vi "RT-v.vi"() -> ()   [LabVIEW 2013]
uses:
  FreqEstimator.ctl
panel:
  out "theta":sgl(graph)
  in  "Scaling":sgl
  in  "alpha":sgl
  in  "Input":sgl
  in  "stop":bool
  in  "Frequency of Oscillation":sgl
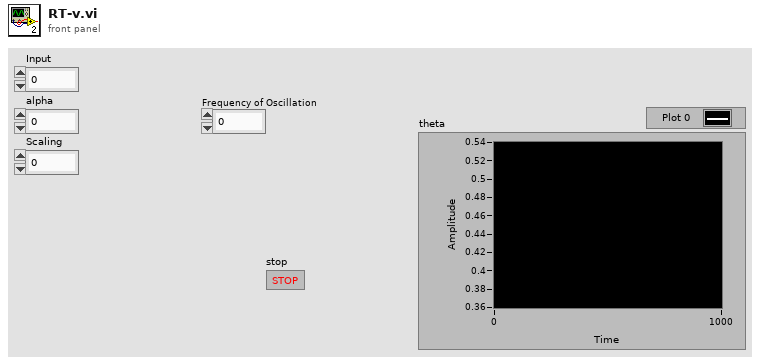
[diagram p1: front panel]
types:
  T1 = typedef "FreqEstimator.ctl" = cluster{"Parameters":cluster{"Ts":sgl, "kappaav":sgl, "kappaph":sgl, "mu":sgl}}
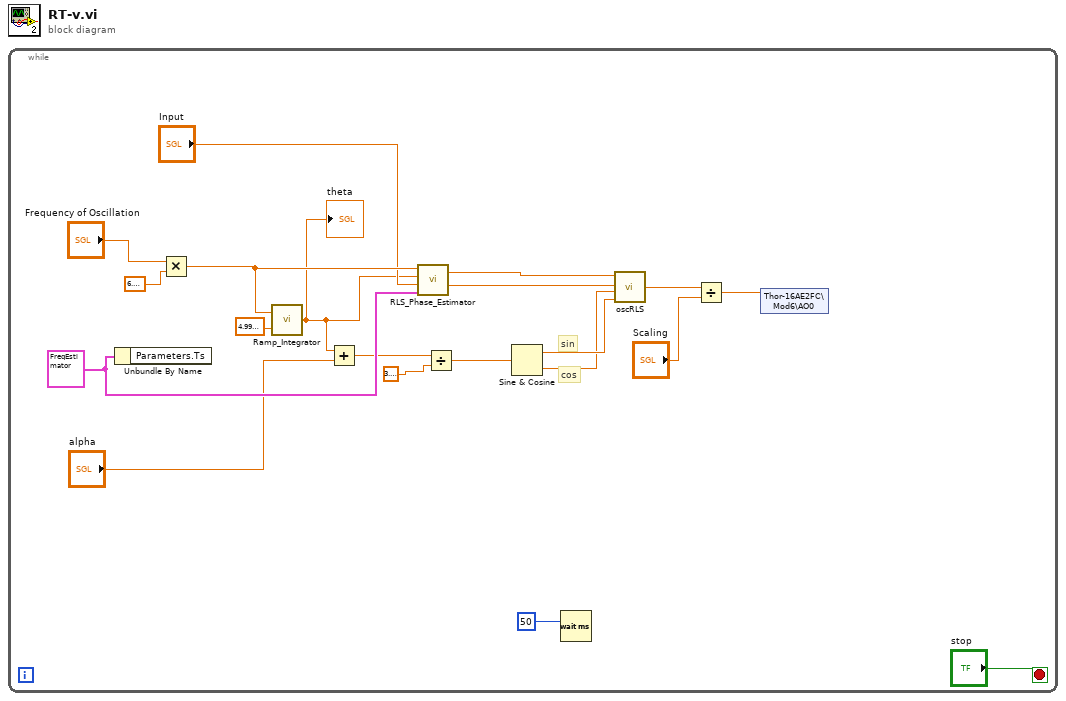
[diagram p0: block diagram]
diagram:
  n1 = while {
    stop <- "stop" stop-if-true
    w14 = T1 {"Parameters"={"Ts"=5e-05, "kappaav"=0.625, "kappaph"=0.5762, "mu"=0.7086}} ("Frequency Estimator Settings")
    # "cos"
    # "sin"
    n2 = Unbundle By Name(w14) -> ()  [unwired: 1 out]
    n3 = Multiply(x="Frequency of Oscillation", y=sgl 6.2831855) -> (x*y=w16:sgl)
    n4 = call "Ramp_Integrator.vi"("tsample"=sgl 5e-05, "w"=w16) -> ("theta"=w11:sgl)
    "theta" <- w11
    n5 = Add(x=w11, y="alpha") -> (x+y=w9:sgl)
    n6 = call "RLS_Phase_Estimator.vi"("Frequency Estimator Settings"=w14, "u"="Input", "theta"=w11, "wcs"=w16) -> ("uphq"=w12:sgl, "uphd"=w13:sgl)
    n7 = Divide(x=w9, y=3.141592653589793) -> (x/y=w7:dbl)
    n8 = Sine & Cosine(0:w7) -> (1:w6:dbl, 2:w5:dbl)
    n9 = Wait (ms)(milliseconds to wait=u32 50) -> ()  [unwired: 1 out]
    n10 = call "oscRLS.vi"("u4"=w6, "u3"=w5, "u2"=w12, "u1"=w13) -> ("f(u)"=w4:sgl)
    n11 = Divide(x=w4, y="Scaling") -> (x/y=w2:sgl)
    n12 = shared-variable "Thor-16AE2FC\\Mod6\\AO0"(w2) -> ()  [unwired: 1 in, 1 out]
  }
